vi "Append Array Element.vi"(4 "JSON Value in":refnum<class "JSON Value.lvclass">, 5 "JSON Value in":refnum<class "JSON Value.lvclass">) -> (1 "JSON Value out":refnum<class "JSON Value.lvclass">)   [LabVIEW 2016, in "JSON Value.lvclass"]
doc: "Appends an array element to an existing JSON Array"
uses:
  JSON Helper/JSON Value.lvclass
  JSON Helper/JSON Value.lvclass/JSON Value.ctl
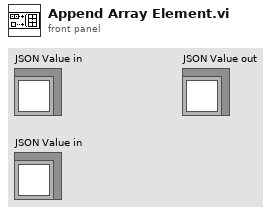
[diagram p1: front panel]
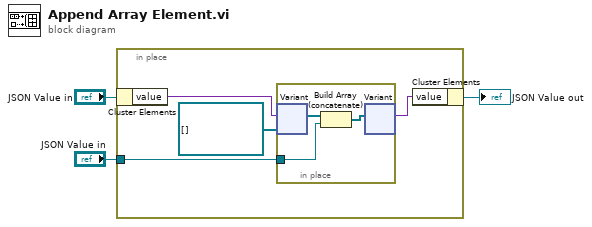
[diagram p0: block diagram]
diagram:
  n1 = in-place {
    in-place-border: "JSON Value in" -> [w7]
    n2 = in-place-cluster #1("JSON Value in") -> ("value"=w6:variant)
    n3 = in-place {
      in-place-border: w7 -> [w10]
      n4 = in-place-variant #2(w6, refnum<class "JSON Value.lvclass">[] [] ("JSON Array in")) -> (w9:refnum<class "JSON Value.lvclass">[])  [unwired: 1 out]
      n5 = Build Array (concatenate)(w9, w10) -> (w8:refnum<class "JSON Value.lvclass">[])
      n6 = in-place-variant #2(w8) -> (w4:variant)  [unwired: 1 out]
    }
    n7 = in-place-cluster #1("value"=w4) -> (→"JSON Value out":refnum<class "JSON Value.lvclass">)
  }
